vi "Row_GetAttributes.vi"(8 "error in (no error)":errorcluster, 10 "OnlyGetDvrReference(False)":bool, 11 "reference in":refnum<class "Row.lvclass">) -> (0 "error out":errorcluster, 1 "DataRef":refnum<data-value>, 2 "Data":T1, 3 "reference out":refnum<class "Row.lvclass">)   [LabVIEW 2012, in "Row.lvclass"]
uses:
  Row.lvclass
  protected/ObjectAttributes.ctl
  Character_class/Character.lvclass
  Glyph_class/Position.ctl
  Row.lvclass/Row.ctl
  Glyph_class/Glyph.lvclass
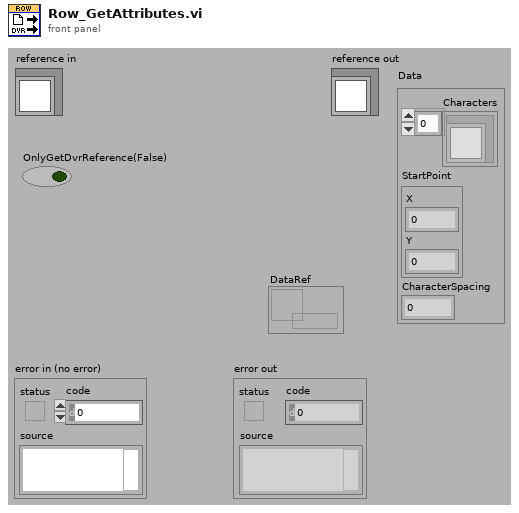
[diagram p1: front panel]
types:
  T1 = typedef "Row.lvclass/ObjectAttributes.ctl" = cluster{"Characters":refnum<class "Character.lvclass">[], "StartPoint":T2, "CharacterSpacing":i32}
  T2 = typedef "Glyph.lvclass/Position.ctl" = cluster{"X":i32, "Y":i32}
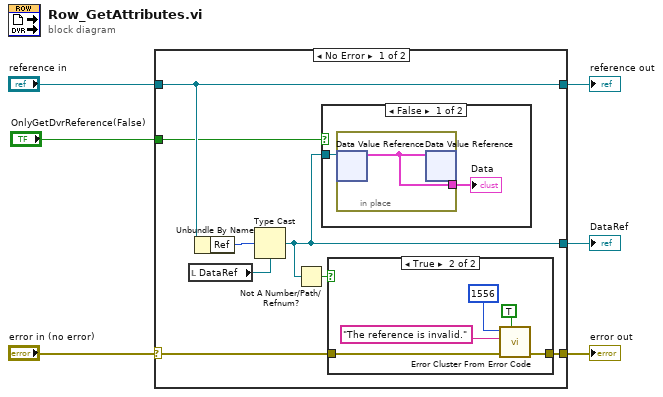
[diagram p0: block diagram]
diagram:
  n1 = case shown="No Error" "error in (no error)" {
    selector: "error in (no error)" -> [w9 w24]
    tunnel: [w8 w24] -> w5
    tunnel: [w14 w25] -> w3
    tunnel: "reference in" -> [w14 w25]
    tunnel: [w10 _] -> w2
    tunnel: "OnlyGetDvrReference(False)" -> [w11 _]
    frame No Error {
      n2 = local read "DataRef"() -> (w12:refnum<data-value>)
      n3 = Unbundle By Name(w14) -> ("Ref"=w13:u32)
      n4 = Type Cast(type=w12, x=w13) -> (*(type *) &x=w10:refnum<data-value>)
      n5 = Not A Number/Path/Refnum?(number/path/refnum=w10) -> (NaN/Path/Refnum?=w7:bool)
      n6 = case shown="False" w11 {
        tunnel: w10 -> [w22 _]
        frame False {
          n7 = in-place {
            in-place-border: [w23] -> w21
            n8 = in-place-dvr #1(w22) -> (w23:T1)  [unwired: 1 out]
            n9 = in-place-dvr #1(w23) -> ()  [unwired: 2 out]
          }
          "Data" <- w21
        }
        frame True {
        }
      }
      n10 = case shown="True" w7 {
        tunnel: w9 -> [w15 w17]
        tunnel: [w15 w16] -> w8
        frame False {
        }
        frame True {
          n11 = call <vilib>:"Error Cluster From Error Code.vi"("show call chain? (False)"=TRUE, "error in (no error)"=w17, "error message (\"\")"="The reference is invalid." ("source"), "error code (0)"=1556 ("code")) -> ("error out"=w16:errorcluster)  [unwired: 5 in]
        }
      }
    }
    frame Error {
    }
  }
  "error out" <- w5
  "reference out" <- w3
  "DataRef" <- w2
